vi "Initialize Kinect.vi"() -> (1 "output cluster":T1, 2 "Error Out":errorcluster)   [LabVIEW 2011]
uses:
  <vilib>/vision/Image Controls.llb/IMAQ Image.ctl
  Microsoft.Kinect
panel:
  in  "Buffer Size 2":i32=10
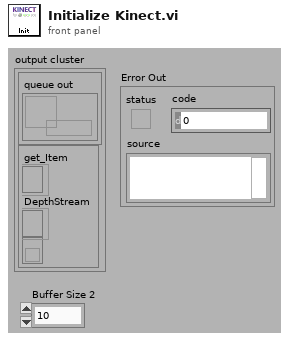
[diagram p1: front panel]
types:
  T1 = cluster{cluster{"queue out":refnum<queue>}, cluster{"get_Item":refnum<k24>, "DepthStream":refnum<k24>, "Event Callback":refnum<k27>}}
  T2 = typedef "IMAQ Image.ctl" = refnum<image>
  T3 = cluster{"get_Item":refnum<k24>, "DepthStream":refnum<k24>, refnum<k27>}
  T4 = cluster{cluster{"queue out":refnum<queue>}, cluster{"get_Item":refnum<k24>, "DepthStream":refnum<k24>, refnum<k27>}}
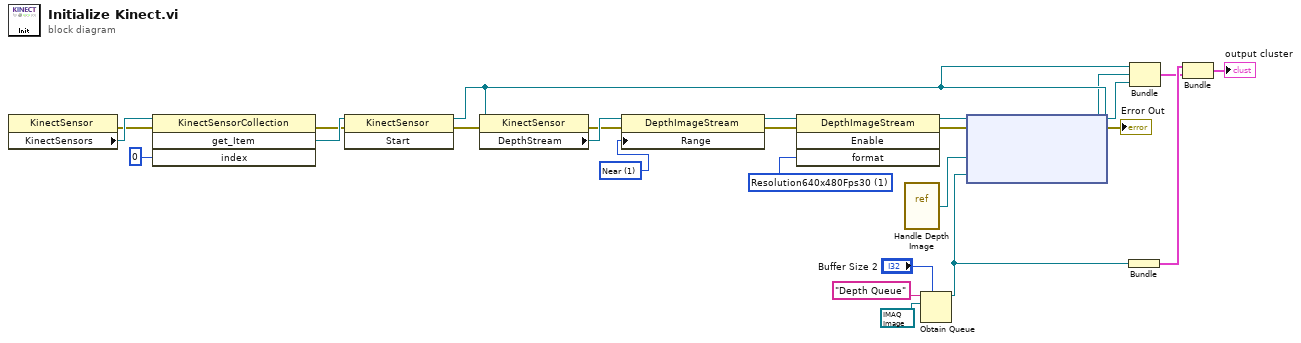
[diagram p0: block diagram]
diagram:
  w4 = 1 items=["Default", "Near"] ("Range")
  w20 = 1 items=["Undefined", "Resolution640x480Fps30", "Resolution320x240Fps30", "Resolution80x60Fps30"] ("format")
  n1 = property class="KinectSensor"() -> (error out=w24:errorcluster, "KinectSensors"=w25:refnum<k24>)  [unwired: 2 in, 1 out]
  n2 = invoke class="KinectSensorCollection" method="get_Item"(reference=w25, error in=w24, "index"=0) -> (error out=w21:errorcluster, "get_Item"=w22:refnum<k24>)  [unwired: 1 in, 2 out]
  n3 = invoke class="KinectSensor" method="Start"(reference=w22, error in=w21) -> (reference out=w7:refnum<k24>, error out=w8:errorcluster)  [unwired: 1 in, 1 out]
  n4 = property class="KinectSensor"(reference=w7, error in=w8) -> (error out=w2:errorcluster, "DepthStream"=w5:refnum<k24>)  [unwired: 1 out]
  n5 = property class="DepthImageStream"(reference=w5, error in=w2, "Range"=w4) -> (reference out=w3:refnum<k24>, error out=w1:errorcluster)
  n6 = invoke class="DepthImageStream" method="Enable"(reference=w3, error in=w1, "format"=w20) -> (reference out=w6:refnum<k24>, error out=w11:errorcluster)  [unwired: 1 in, 2 out]
  n7 = vi-ref "Handle Depth Image.vi"() -> (w12:refnum<vi>)
  n8 = Obtain Queue(max queue size (-1, unlimited)="Buffer Size 2", name (unnamed)="Depth Queue", element data type=T2 refnum ("New Image")) -> (queue out=w16:refnum<queue>)  [unwired: 2 in, 2 out]
  n9 = node(w11, w7, w12, w16) -> (w10:refnum<k27>, →"Error Out":errorcluster)  [unwired: 1 in]
  n10 = Bundle("queue out"=w16) -> (w15:cluster{"queue out":refnum<queue>})  [unwired: 1 in]
  n11 = Bundle("get_Item"=w7, "DepthStream"=w6, w10) -> (w14:T3)  [unwired: 1 in]
  n12 = Bundle(w15, w14) -> (→"output cluster":T4)  [unwired: 1 in]
